vi "Init Device.vi"(7 "Layout Ref":refnum<vi>, 8 "error in (no error)":errorcluster, 10 "Chan# Array":i32[](array[numeric]), 11 "TestMenu in":refnum<class "TestMenu.lvclass">) -> (0 "error out":errorcluster, 3 "TestMenu out":refnum<class "TestMenu.lvclass">)   [LabVIEW 2013, in "TestMenu.lvclass"]
doc: "Initialize the correct columns and their default appearance.\nUse the front panel to change default appearance of the device in the Add/Manage devices.\n\nOpen a specific device implementation for details."
uses:
  TestMenu.lvclass
  ColumnVIs/MenuCol/MenuCol.lvclass
  ColumnVIs/SingleValMenuCol/SingleValMenuCol.lvclass
  ColumnVIs/MenuDisableCol/MenuDisableCol.lvclass
  TypeDefs/ColumnAppearCluster.ctl
  ColumnVIs/MenuDisableCol/MenuItemDisables.ctl
  ColumnVIs/Column/Column.lvclass
panel:
  in  "Those Column that disable the other ones":T1[](array[typedef])=[{"MenuEntry"="None", "DisableColumns"=[]}, {"MenuEntry"="-2", "DisableColumns"=[-2]}, {"MenuEntry"="-1, -3", "DisableColumns"=[-1, -3]}]
  in  "Disable Appearance":T2={"Column Name"="Variables!", "Width"=30, "Bkgd"=[16752889], "Text"=[0]}
  in  "Single Val Appearance":T2={"Column Name"="No Variables!", "Width"=30, "Bkgd"=[16774656], "Text"=[0]}
  in  "No Variable Appearance":T2={"Column Name"="No Variables!", "Width"=30, "Bkgd"=[16753962], "Text"=[0]}
  in  "MenuItemList":string[](array[string])=["Item 0", "Item 1", "Some sort of long-winded item"]
  in  "Variable Appearance":T2={"Column Name"="Variables!", "Width"=30, "Bkgd"=[4375295, 7471101], "Text"=[0]}
  in  "Device Description":string="A dummy device designed only to test the operation of a Menu Column"
  in  "Name":string="Test Menu Column"
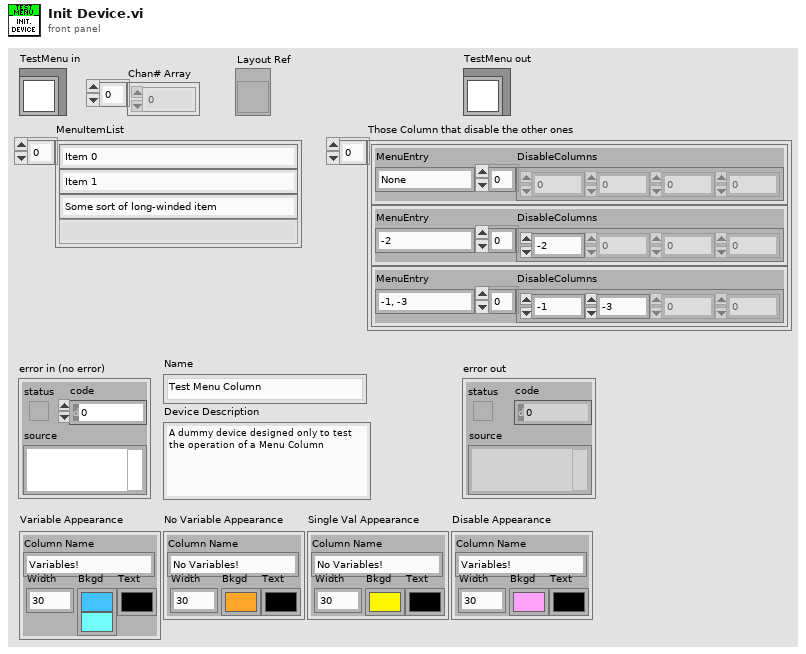
[diagram p1: front panel]
types:
  T1 = typedef "MenuItemDisables.ctl" = cluster{"MenuEntry":string, "DisableColumns":i32[]}
  T2 = typedef "ColumnAppearCluster.ctl" = cluster{"Column Name":string, "Width":u32, "Bkgd":u32[], "Text":u32[]}
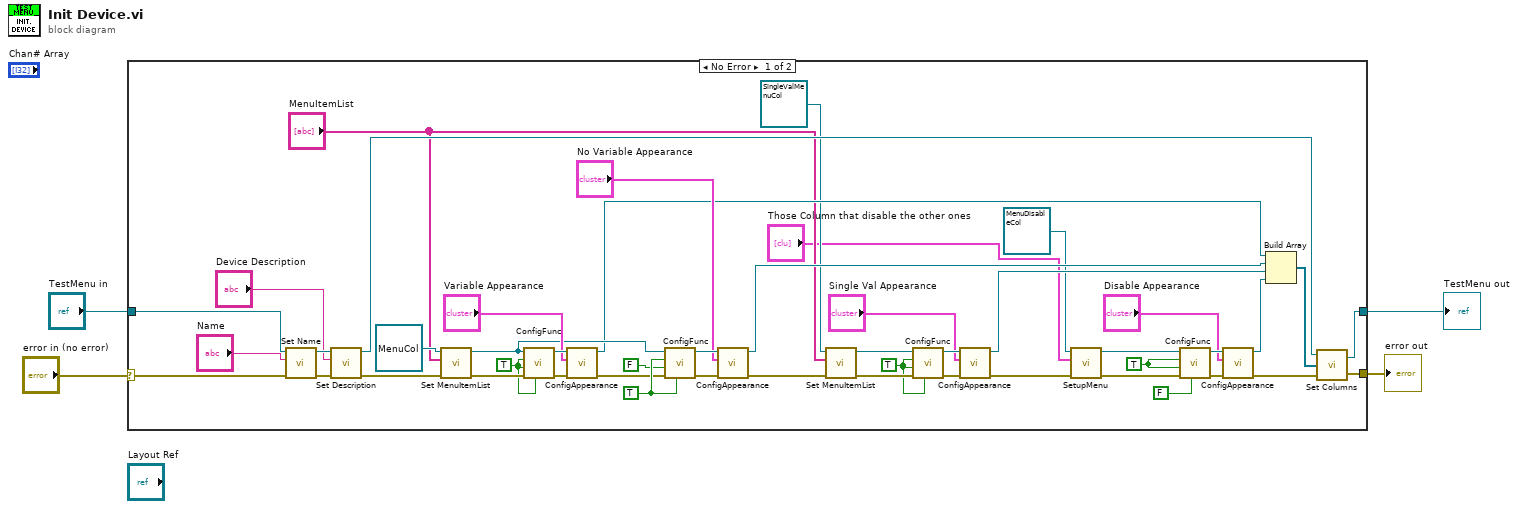
[diagram p0: block diagram]
diagram:
  n1 = case shown="No Error" "error in (no error)" {
    selector: "error in (no error)" -> [w48 w54]
    tunnel: [w46 w54] -> w3
    tunnel: "TestMenu in" -> [w52 w53]
    tunnel: [w45 w53] -> w1
    frame No Error {
      w8 = TRUE ("Disableable? (True)")
      w19 = TRUE ("isVariable? (True)")
      w33 = TRUE ("isRampable? (True")
      w38 = TRUE ("isVariable? (True)")
      n2 = call-dynamic "Set Name.vi"("error in (no error)"=w48, "Name"="Name", "Device in"=w52) -> ("error out"=w47:errorcluster, "Device out"=w51:refnum<class "TestMenu.lvclass">)  [unwired: 7 in]
      n3 = call-dynamic "Set Description.vi"("error in (no error)"=w47, "Device Description"="Device Description", "Device in"=w51) -> ("error out"=w40:errorcluster, "Device out"=w44:refnum<class "TestMenu.lvclass">)  [unwired: 7 in]
      n4 = call-dynamic "Set MenuItemList.vi"("error in (no error)"=w40, "MenuItemList"="MenuItemList", "MenuCol in"=refnum<class "MenuCol.lvclass"> refnum ("MenuCol.lvclass")) -> ("error out"=w39:errorcluster, "MenuCol out"=w31:refnum<class "MenuCol.lvclass">)  [unwired: 7 in]
      n5 = call "ConfigFunc.vi"("isRampable? (True"=w38, "error in (no error)"=w39, "isVariable? (True)"=w38, "Disableable? (True)"=w38, "Column in"=w31) -> ("error out"=w43:errorcluster, "Column out"=w42:refnum<class "MenuCol.lvclass">)  [unwired: 5 in]
      n6 = call "ConfigAppearance.vi"("error in (no error)"=w43, "Column Appearance"="Variable Appearance", "Column in"=w42) -> ("error out"=w30:errorcluster, "Column out"=w29:refnum<class "MenuCol.lvclass">)  [unwired: 7 in]
      n7 = call "ConfigFunc.vi"("isRampable? (True"=w33, "error in (no error)"=w30, "isVariable? (True)"=FALSE, "Disableable? (True)"=w33, "Column in"=w31) -> ("error out"=w37:errorcluster, "Column out"=w36:refnum<class "MenuCol.lvclass">)  [unwired: 5 in]
      n8 = call "ConfigAppearance.vi"("error in (no error)"=w37, "Column Appearance"="No Variable Appearance", "Column in"=w36) -> ("error out"=w20:errorcluster, "Column out"=w28:refnum<class "MenuCol.lvclass">)  [unwired: 7 in]
      n9 = call-dynamic "Set MenuItemList.vi"("error in (no error)"=w20, "MenuItemList"="MenuItemList", "MenuCol in"=refnum<class "SingleValMenuCol.lvclass"> refnum ("SingleValMenuCol.lvclass")) -> ("error out"=w25:errorcluster, "MenuCol out"=w26:refnum<class "SingleValMenuCol.lvclass">)  [unwired: 7 in]
      n10 = call "ConfigFunc.vi"("isRampable? (True"=w19, "error in (no error)"=w25, "isVariable? (True)"=w19, "Disableable? (True)"=w19, "Column in"=w26) -> ("error out"=w23:errorcluster, "Column out"=w24:refnum<class "SingleValMenuCol.lvclass">)  [unwired: 5 in]
      n11 = call "ConfigAppearance.vi"("error in (no error)"=w23, "Column Appearance"="Single Val Appearance", "Column in"=w24) -> ("error out"=w5:errorcluster, "Column out"=w18:refnum<class "SingleValMenuCol.lvclass">)  [unwired: 7 in]
      n12 = call-dynamic "SetupMenu.vi"("error in (no error)"=w5, "MenuItemDisablesList"="Those Column that disable the other ones", "MenuDisableCol in"=refnum<class "MenuDisableCol.lvclass"> refnum ("MenuDisableCol.lvclass")) -> ("error out"=w14:errorcluster, "MenuDisableCol out"=w12:refnum<class "MenuDisableCol.lvclass">)  [unwired: 7 in]
      n13 = call "ConfigFunc.vi"("isRampable? (True"=FALSE, "error in (no error)"=w14, "isVariable? (True)"=w8, "Disableable? (True)"=w8, "Column in"=w12) -> ("error out"=w13:errorcluster, "Column out"=w11:refnum<class "MenuDisableCol.lvclass">)  [unwired: 5 in]
      n14 = call "ConfigAppearance.vi"("error in (no error)"=w13, "Column Appearance"="Disable Appearance", "Column in"=w11) -> ("error out"=w6:errorcluster, "Column out"=w7:refnum<class "MenuDisableCol.lvclass">)  [unwired: 7 in]
      n15 = Build Array(w29, w28, w18, w7) -> (w27:refnum<class "MenuCol.lvclass">[])
      n16 = call-dynamic "Set Columns.vi"("error in (no error)"=w6, "Columns"=w27, "Device in"=w44) -> ("error out"=w46:errorcluster, "Device out"=w45:refnum<class "TestMenu.lvclass">)  [unwired: 1 in]
    }
    frame Error {
    }
  }
  "error out" <- w3
  "TestMenu out" <- w1
